vi "Click2CursorPosition.vi"(0 "reference":refnum<vi>, 7 "ClickPosition":T1) -> (6 "CursorX":dbl, 10 "CursorY":dbl)   [LabVIEW 2011]
uses:
  <vilib>/Utility/miscctls.llb/LVPoint32TypeDef.ctl
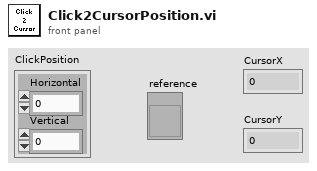
[diagram p1: front panel]
types:
  T1 = typedef "LVPoint32TypeDef.ctl" = cluster{"Horizontal":i32, "Vertical":i32}
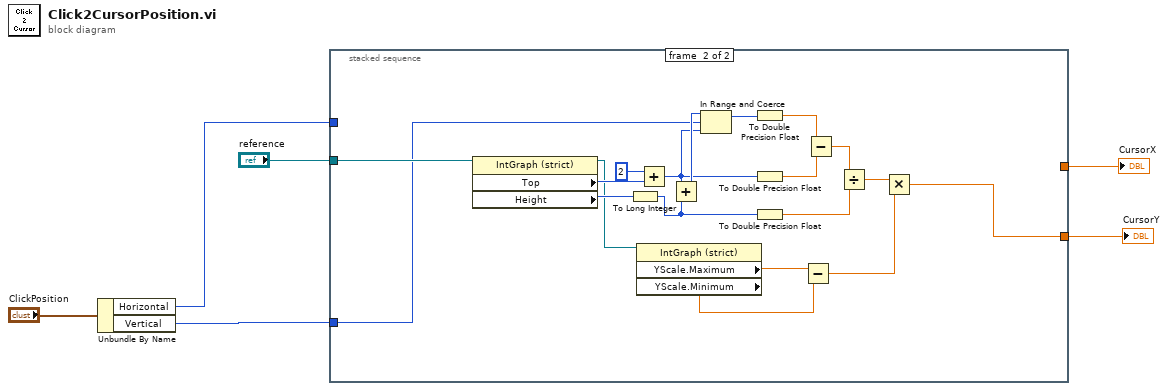
[diagram p0: block diagram]
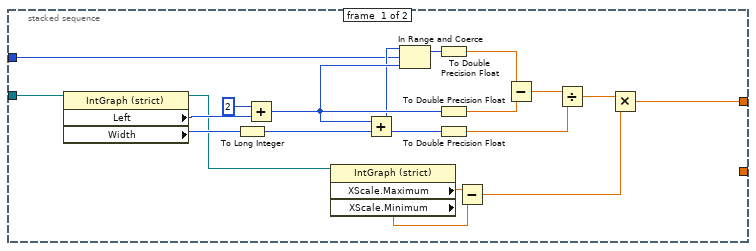
[diagram p2: hidden frame]
diagram:
  n1 = Unbundle By Name("ClickPosition") -> ("Horizontal"=w2:i32, "Vertical"=w1:i32)
  n2 = stacked-sequence {
    tunnel: [w19 _] -> w6
    tunnel: "reference" -> [w9 w29]
    tunnel: [_ w26] -> w3
    tunnel: w2 -> [w7 _]
    tunnel: w1 -> [_ w28]
    frame #0 {
      n3 = property on="Property Node" class="IntGraph (strict)"(reference=w9) -> (reference out=w8:refnum<vi>, "Left"=w24:i32, "Width"=w25:u32)  [unwired: 1 in, 1 out]
      n4 = To Long Integer(number=w25) -> (32bit integer=w12:i32)
      n5 = Add(x=2, y=w24) -> (x+y=w21:i32)
      n6 = property on="Property Node" class="IntGraph (strict)"(reference=w8) -> ("XScale.Maximum"=w16:dbl, "XScale.Minimum"=w17:dbl)  [unwired: 1 in, 2 out]
      n7 = Add(x=w21, y=w12) -> (x+y=w11:i32)
      n8 = In Range and Coerce(upper limit=w11, x=w7, lower limit=w21) -> (coerced(x)=w13:i32)  [unwired: 1 out]
      n9 = To Double Precision Float(number=w13) -> (double precision float=w20:dbl)
      n10 = To Double Precision Float(number=w21) -> (double precision float=w22:dbl)
      n11 = To Double Precision Float(number=w12) -> (double precision float=w14:dbl)
      n12 = Subtract(x=w16, y=w17) -> (x-y=w18:dbl)
      n13 = Subtract(x=w20, y=w22) -> (x-y=w23:dbl)
      n14 = Divide(x=w23, y=w14) -> (x/y=w15:dbl)
      n15 = Multiply(x=w15, y=w18) -> (x*y=w19:dbl)
    }
    frame #1 {
      n16 = property on="Property Node" class="IntGraph (strict)"(reference=w29) -> (reference out=w27:refnum<vi>, "Top"=w32:i32, "Height"=w31:u32)  [unwired: 1 in, 1 out]
      n17 = To Long Integer(number=w31) -> (32bit integer=w36:i32)
      n18 = property on="Property Node" class="IntGraph (strict)"(reference=w27) -> ("YScale.Maximum"=w44:dbl, "YScale.Minimum"=w40:dbl)  [unwired: 1 in, 2 out]
      n19 = Add(x=2, y=w32) -> (x+y=w34:i32)
      n20 = Add(x=w34, y=w36) -> (x+y=w42:i32)
      n21 = In Range and Coerce(upper limit=w42, x=w28, lower limit=w34) -> (coerced(x)=w37:i32)  [unwired: 1 out]
      n22 = To Double Precision Float(number=w37) -> (double precision float=w33:dbl)
      n23 = To Double Precision Float(number=w34) -> (double precision float=w35:dbl)
      n24 = To Double Precision Float(number=w36) -> (double precision float=w38:dbl)
      n25 = Subtract(x=w44, y=w40) -> (x-y=w41:dbl)
      n26 = Subtract(x=w33, y=w35) -> (x-y=w30:dbl)
      n27 = Divide(x=w30, y=w38) -> (x/y=w39:dbl)
      n28 = Multiply(x=w39, y=w41) -> (x*y=w26:dbl)
    }
  }
  "CursorX" <- w6
  "CursorY" <- w3
